vi "GetIndexNum_Arithmatic.vi"(0 "ArrayRef":refnum<vi>, 11 "error in (no error)":errorcluster) -> (4 "ArrayRef out":refnum<vi>, 6 "ItemIndex":T1, 15 "error out":errorcluster)   [LabVIEW 2009]
doc: "To get the index number of the item in a 2D array when you click. \nMake sure the 2D array have no visible item, or there will be some arithemic mistakes.\nIf the 2D array have visible items, use GetIndexNum.vi \n\nThis VI is written by Cai Zhibin.\n------------------------------------\nArrayRef: Reference of the 2D array.\nArrayRef out: Pass out the reference.\nItemIndex_row: The Result number (row).\nItemIndex_col: The Result number (column).\nerror in(no error): Error cluster passed in.\nerror out: Pass out the error cluster."
uses:
  Controls/ItemIndex.ctl
panel:
  in  "ItemIndex1":T1
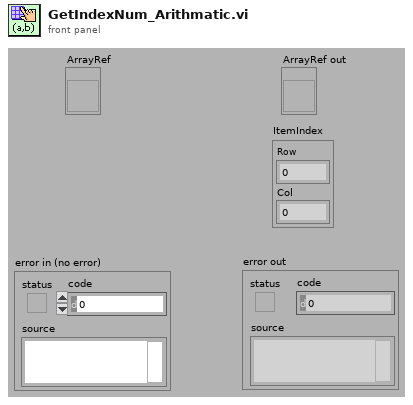
[diagram p1: front panel]
types:
  T1 = typedef "ItemIndex.ctl" = cluster{"Row":i32, "Col":i32}
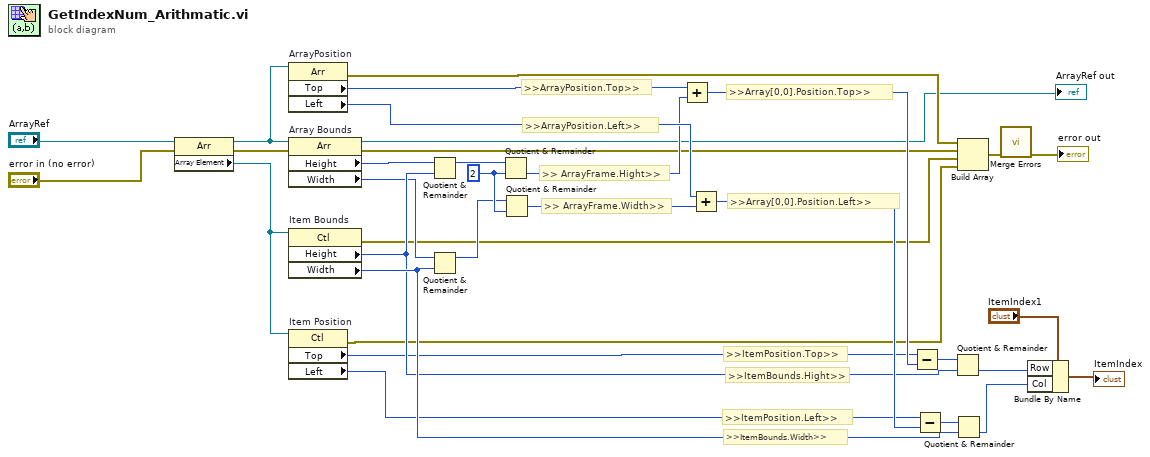
[diagram p0: block diagram]
diagram:
  w22 = u32 2 ("y")
  # ">>ItemBounds.Width>>"
  # ">>ItemBounds.Hight>>"
  # ">>ItemPosition.Left>>"
  # ">>ItemPosition.Top>>"
  # ">>ArrayPosition.Left>>"
  # ">>ArrayPosition.Top>>"
  # ">>Array[0,0].Position.Left>>"
  # ">>Array[0,0].Position.Top>>"
  # ">> ArrayFrame.Width>>"
  # ">> ArrayFrame.Hight>>"
  n1 = property class="Arr"(reference="ArrayRef", error in="error in (no error)") -> (reference out=w18:refnum<vi>, error out=w13:errorcluster, "Array Element"=w25:refnum<vi>)
  n2 = property on="ArrayPosition" class="Arr"(reference=w18) -> (error out=w12:errorcluster, "Top"=w19:i32, "Left"=w24:i32)  [unwired: 1 in, 1 out]
  n3 = property on="Array Bounds" class="Arr"(reference=w18, error in=w13) -> (reference out=→"ArrayRef out":refnum<vi>, error out=w11:errorcluster, "Height"=w15:u32, "Width"=w16:u32)
  n4 = property on="Item Bounds" class="Ctl"(reference=w25) -> (error out=w10:errorcluster, "Height"=w29:u32, "Width"=w33:u32)  [unwired: 1 in, 1 out]
  n5 = property on="Item Position" class="Ctl"(reference=w25) -> (error out=w9:errorcluster, "Top"=w26:i32, "Left"=w31:i32)  [unwired: 1 in, 1 out]
  n6 = Quotient & Remainder(x=w15, y=w29) -> (x-y*floor(x/y)=w17:u32)  [unwired: 1 out]
  n7 = Quotient & Remainder(x=w16, y=w33) -> (x-y*floor(x/y)=w21:u32)  [unwired: 1 out]
  n8 = Quotient & Remainder(x=w17, y=w22) -> (floor(x/y)=w20:u32)  [unwired: 1 out]
  n9 = Quotient & Remainder(x=w21, y=w22) -> (floor(x/y)=w23:u32)  [unwired: 1 out]
  n10 = Add(x=w19, y=w20) -> (x+y=w27:u32)
  n11 = Add(x=w24, y=w23) -> (x+y=w32:u32)
  n12 = Subtract(x=w26, y=w27) -> (x-y=w28:u32)
  n13 = Subtract(x=w31, y=w32) -> (x-y=w30:u32)
  n14 = Quotient & Remainder(x=w28, y=w29) -> (floor(x/y)=w3:u32)  [unwired: 1 out]
  n15 = Quotient & Remainder(x=w30, y=w33) -> (floor(x/y)=w2:u32)  [unwired: 1 out]
  n16 = Build Array(w12, w11, w10, w9) -> (w8:errorcluster[])
  n17 = call <vilib>:"Merge Errors.vi"("error array in"=w8) -> ("error out"=→"error out":errorcluster)  [unwired: 6 in]
  n18 = Bundle By Name(cluster="ItemIndex1", "Row"=w3, "Col"=w2) -> (→"ItemIndex":T1)
